vi "Latch.vi"(0 "Input":bool, 1 "reset":bool) -> (4 "Output":bool)   [LabVIEW 2014]
doc: "This VI latches an input until the reset signal is recieved :i.e. When input is asserted, output is asserted until the reset signal is raised."
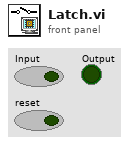
[diagram p1: front panel]
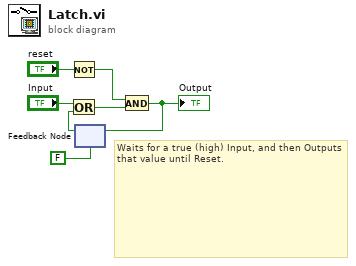
[diagram p0: block diagram]
diagram:
  # "Waits for a true (high) Input, and then Outputs that value until Reset."
  n1 = Not(x="reset") -> (.not. x?=w2:bool)
  n2 = feedback #1(FALSE) -> (w6:bool)
  n3 = Or(x="Input", y=w6) -> (x .or. y?=w4:bool)
  n4 = And(x=w2, y=w4) -> (x .and. y?=w7:bool)
  "Output" <- w7
  n5 = feedback-in #1(w7) -> ()
